vi "Read Measurement.vi"(8 "error in (no error)":errorcluster, 10 "Vin SMU Channel":string, 11 "IVI Refnum in":refnum<k15>) -> (0 "error out":errorcluster, 2 "Current":dbl, 3 "Voltage":dbl)   [LabVIEW 2021, in "SMU T11.lvlib"]
uses:
  SMU T11.lvlib
  <instrlib>/niDCPower/nidcpower.llb/niDCPower Wait For Event - Event.ctl
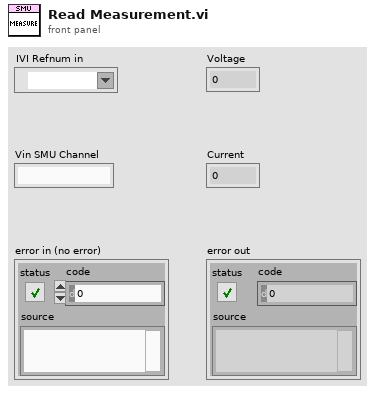
[diagram p1: front panel]
types:
  T1 = typedef "niDCPower Wait For Event - Event.ctl" = i32
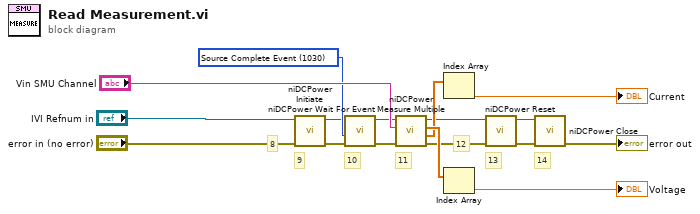
[diagram p0: block diagram]
diagram:
  w9 = T1 1030 items=["Source Complete Event"=1030, "Measure Complete Event"=1031, "Sequence Iteration Complete Event"=1032, "Sequence Engine Done Event"=1033] ("event")
  # "14"
  # "9"
  # "11"
  # "10"
  # "12"
  # "13"
  # "8"
  n1 = call <instrlib>:"niDCPower Initiate.vi"("error in (no error)"="error in (no error)", "instrument handle"="IVI Refnum in") -> ("error out"=w7:errorcluster, "instrument handle out"=w5:refnum<k15>)  [unwired: 2 in, 6 out]
  n2 = call <instrlib>:"niDCPower Wait For Event.vi"("error in (no error)"=w7, "event"=w9, "instrument handle"=w5) -> ("error out"=w8:errorcluster, "instrument handle out"=w6:refnum<k15>)  [unwired: 1 in, 6 out]
  n3 = call <instrlib>:"niDCPower Measure Multiple.vi"("error in (no error)"=w8, "channel name"="Vin SMU Channel", "instrument handle"=w6) -> ("error out"=w4:errorcluster, "current measurements"=w10:dbl[], "voltage measurements"=w11:dbl[], "instrument handle out"=w3:refnum<k15>)  [unwired: 5 out]
  n4 = Index Array(array=w10) -> (element=→"Current":dbl)  [unwired: 1 in]
  n5 = Index Array(array=w11) -> (element=→"Voltage":dbl)  [unwired: 1 in]
  n6 = call <instrlib>:"niDCPower Reset.vi"("error in (no error)"=w4, "instrument handle"=w3) -> ("error out"=w2:errorcluster, "instrument handle out"=w1:refnum<k15>)  [unwired: 2 in, 6 out]
  n7 = call <instrlib>:"niDCPower Close.vi"("error in (no error)"=w2, "instrument handle"=w1) -> ("error out"=→"error out":errorcluster)  [unwired: 9 out]
